vi "generator.vi"() -> ()   [LabVIEW 2009]
uses:
  <vilib>/measure/madcrms.llb/Basic Averaged DC-RMS for N Chan.vi
  <vilib>/measure/matone.llb/Extract Single Tone Information N Chan.vi
  <vilib>/Utility/file.llb/Write To Spreadsheet File (DBL).vi
  <vilib>/measure/NI_MAPro.lvlib
  <vilib>/Analysis/NI_AALPro.lvlib
panel:
  out "Fuel GPM":dbl
  in  "Clear Data":bool
  in  "Record Data":bool
  in  "Save Data To CSV?":bool
  in  "CSV Save Path":path
  in  "Append?":bool
  out "Shop Water\nFlow (GPM)":dbl
  out "Jacket \nWater\nFlow\n(GPM)":dbl
  out "Exhaust Temp. (F)":dbl
  out "Shop\nWater\nOut (F)":dbl
  out "Shop\nWater\nIn (F)":dbl
  out "Jacket\nWater\nOut (F)":dbl
  out "Jacket \nWater\nIn (F)":dbl
  out "Oil Temp. (F)":dbl
  out "Fuel (gal.)":dbl(slide) scale=0.0..20.0
  out "Load (kW)":dbl format="%.1f"
  in  "?":bool
  # "CSV Headers:\ntime [s],\nT oil [F],\nT jacket in [F] ,\nT jacket out [F],\nT shop in [F],\nT shop out [F],\nT exhaust [F],\nLoad [kW],\nFuel [gal] ,\nShop Flow [GPM],\nJacket Flow [GPM]"
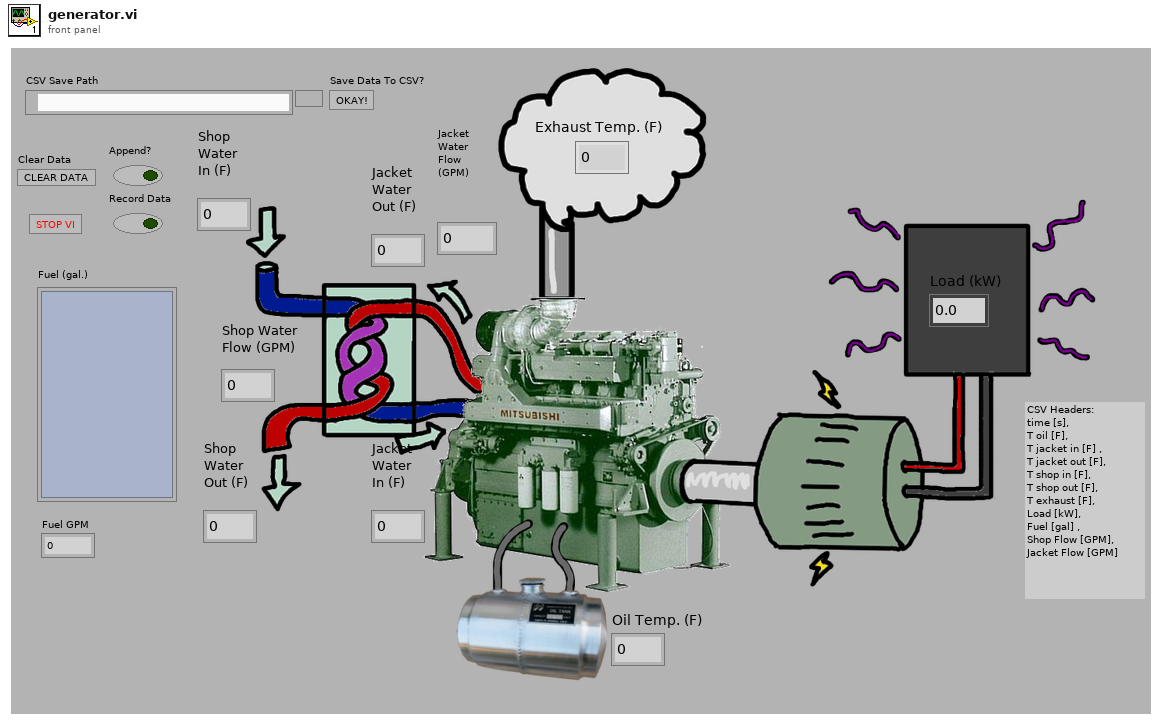
[diagram p1: front panel]
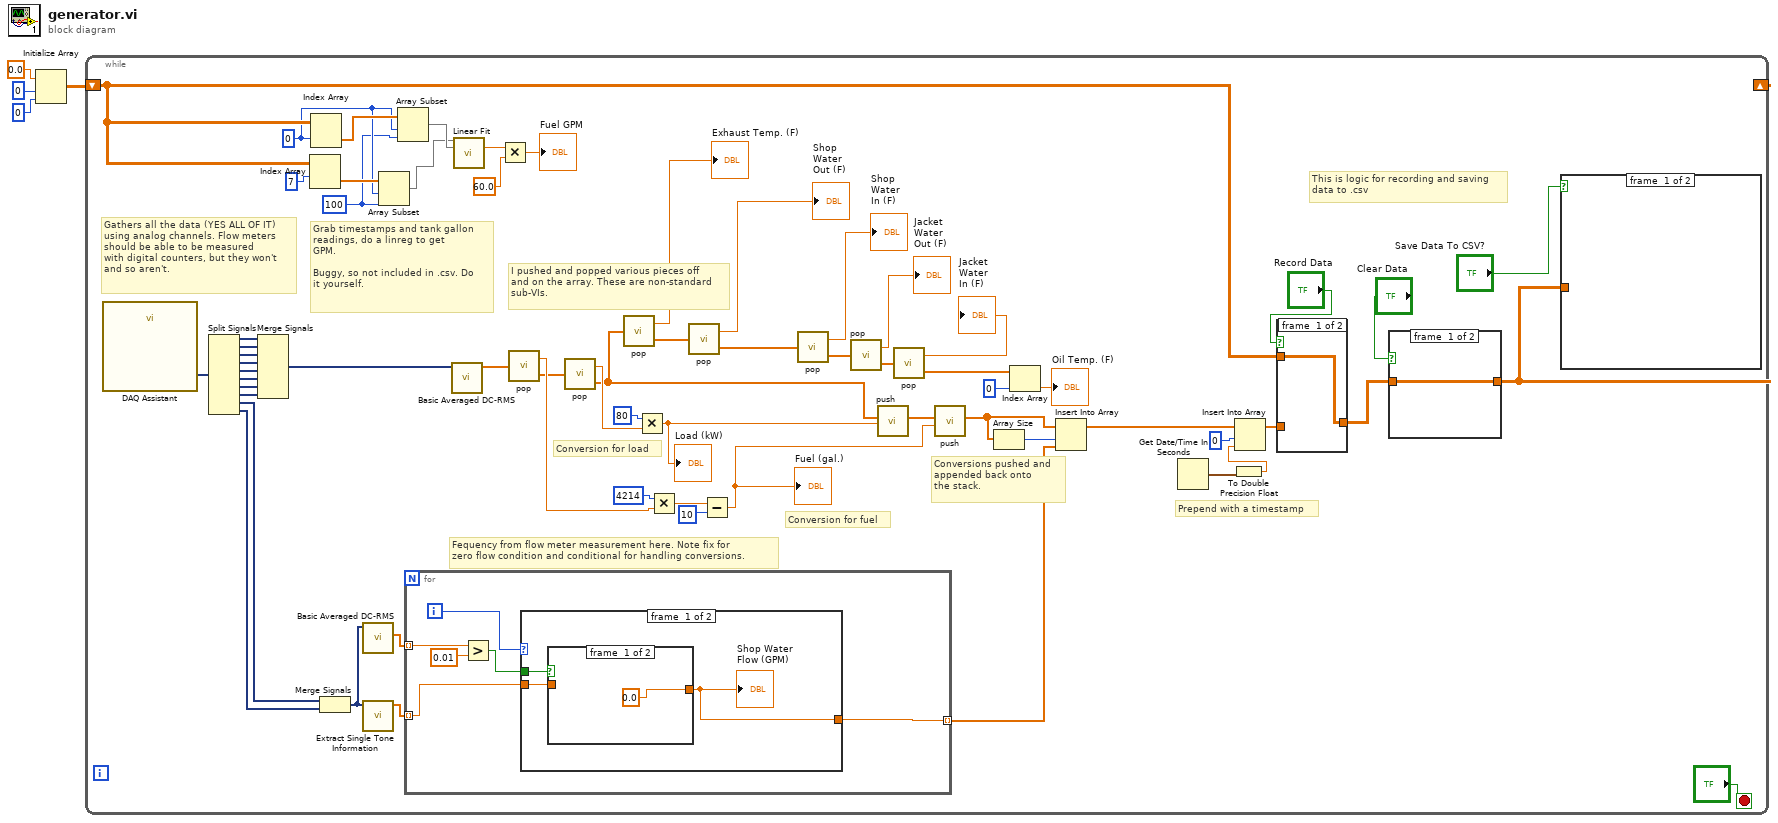
[diagram p0: block diagram]
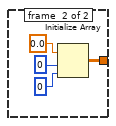
[diagram p2: hidden frame]
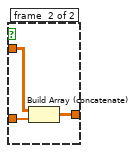
[diagram p3: hidden frame]
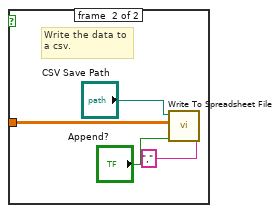
[diagram p4: hidden frame]
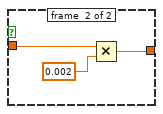
[diagram p5: hidden frame]
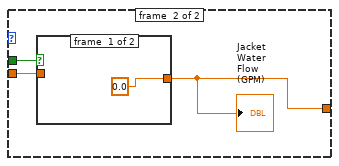
[diagram p6: hidden frame]
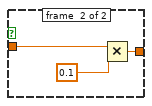
[diagram p7: hidden frame]
diagram:
  n1 = Initialize Array(0.0, 0, 0) -> (w1:dbl[][])
  n2 = while {
    shift-right: [w21] -> _
    shift-left: w1 -> [w16]
    stop <- "?" stop-if-true
    w8 = 100
    w10 = 0
    # "Grab timestamps and tank gallon\nreadings, do a linreg to get\nGPM.\n\nBuggy, so not included in .csv. Do\nit yourself."
    # "This is logic for recording and saving\ndata to .csv"
    # "Conversions pushed and\nappended back onto\nthe stack."
    # "Conversion for fuel"
    # "Conversion for load"
    # "I pushed and popped various pieces off\nand on the array. These are non-standard\nsub-VIs."
    # "Fequency from flow meter measurement here. Note fix for\nzero flow condition and conditional for handling conversions."
    # "Gathers all the data (YES ALL OF IT)\nusing analog channels. Flow meters\nshould be able to be measured\nwith digital counters, but they won't\nand so aren't."
    # "Prepend with a timestamp"
    n3 = call "DAQ Assistant"() -> ("data"=w55:dynamicdata)  [unwired: 17 in, 2 out]
    n4 = Split Signals(w55) -> (w42:dynamicdata, w41:dynamicdata, w40:dynamicdata, w39:dynamicdata, w38:dynamicdata, w37:dynamicdata, w36:dynamicdata, w35:dynamicdata, w34:dynamicdata, w33:dynamicdata)  [unwired: 10 in]
    n5 = Merge Signals(w42, w41, w40, w39, w38, w37, w36, w35) -> (w44:dynamicdata)
    n6 = Index Array(array=w16, index (row)=7) -> (element=w14:dbl[])  [unwired: 1 in]
    n7 = Index Array(array=w16, index (row)=w10) -> (element=w13:dbl[])  [unwired: 1 in]
    n8 = Merge Signals(w34, w33) -> (w43:dynamicdata)
    n9 = call-poly <vilib>:"Basic Averaged DC-RMS.vi"("signals in"=w43) -> ("RMS values"=w45:dbl[])  [unwired: 7 in, 3 out]
    n10 = call-poly <vilib>:"Extract Single Tone Information.vi"("time signals in"=w43) -> ("detected frequencies"=w46:dbl[])  [unwired: 5 in, 5 out]
    n11 = Array Subset(array=w14, index=w10, length=w8) -> (w11:dbl[])
    n12 = Array Subset(array=w13, index=w10, length=w8) -> (w12:dbl[])
    n13 = for {
      tunnel: w46 -> [w82] mode=indexing
      tunnel: w45 -> [w87] mode=indexing
      tunnel: [w84] -> w17 mode=indexing
      i -> [w85]
      n14 = Greater?(x=w87, y=0.01) -> (0:w83:bool)
      n15 = case shown="0, Default" w85 {
        tunnel: [w89 w95] -> w84
        tunnel: w83 -> [w90 w97]
        tunnel: w82 -> [w88 w96]
        frame #0 {
          n16 = case shown="False" w90 {
            tunnel: [0.0 w93] -> w89
            tunnel: w88 -> [_ w92]
            frame #0 {
            }
            frame #1 {
              n17 = Multiply(x=w92, y=0.002) -> (x*y=w93:dbl)
            }
          }
          "Shop Water\nFlow (GPM)" <- w89
        }
        frame #1 {
          n18 = case shown="False" w97 {
            tunnel: [0.0 w100] -> w95
            tunnel: w96 -> [_ w99]
            frame #0 {
            }
            frame #1 {
              n19 = Multiply(x=w99, y=0.1) -> (x*y=w100:dbl)
            }
          }
          "Jacket \nWater\nFlow\n(GPM)" <- w95
        }
      }
    }
    n20 = call-poly <vilib>:"Basic Averaged DC-RMS.vi"("signals in"=w44) -> ("DC values"=w52:dbl[])  [unwired: 7 in, 3 out]
    n21 = call <vilib>:"Linear Fit.vi"("Y"=w11, "X"=w12) -> ("slope"=w6:dbl)  [unwired: 9 in, 4 out]
    n22 = Multiply(x=w6, y=60.0) -> (x*y=→"Fuel GPM":dbl)
    n23 = call "pop.vi"("Before"=w52) -> ("Popped"=w53:dbl, "After"=w51:dbl[])  [unwired: 4 in]
    n24 = call "pop.vi"("Before"=w51) -> ("Popped"=w54:dbl, "After"=w26:dbl[])  [unwired: 4 in]
    n25 = call "pop.vi"("Before"=w26) -> ("Popped"=→"Exhaust Temp. (F)":dbl, "After"=w66:dbl[])  [unwired: 4 in]
    n26 = Multiply(x=80, y=w54) -> (x*y=w25:dbl)
    "Load (kW)" <- w25
    n27 = Multiply(x=4214, y=w53) -> (x*y=w50:dbl)
    n28 = call "pop.vi"("Before"=w66) -> ("Popped"=→"Shop\nWater\nOut (F)":dbl, "After"=w64:dbl[])  [unwired: 4 in]
    n29 = Subtract(x=w50, y=10) -> (x-y=w23:dbl)
    "Fuel (gal.)" <- w23
    n30 = call "pop.vi"("Before"=w64) -> ("Popped"=→"Shop\nWater\nIn (F)":dbl, "After"=w62:dbl[])  [unwired: 4 in]
    n31 = call "pop.vi"("Before"=w62) -> ("Popped"=→"Jacket\nWater\nOut (F)":dbl, "After"=w60:dbl[])  [unwired: 4 in]
    n32 = call "push.vi"("Push"=w25, "Before"=w26) -> ("After"=w24:dbl[])  [unwired: 9 in]
    n33 = call "pop.vi"("Before"=w60) -> ("Popped"=→"Jacket \nWater\nIn (F)":dbl, "After"=w58:dbl[])  [unwired: 4 in]
    n34 = call "push.vi"("Push"=w23, "Before"=w24) -> ("After"=w19:dbl[])  [unwired: 9 in]
    n35 = Array Size(array=w19) -> (size(s)=w18:i32)
    n36 = Index Array(array=w58, index=0) -> (element=→"Oil Temp. (F)":dbl)
    n37 = Insert Into Array(array=w19, index=w18, new element=w17) -> (w5:dbl[])
    n38 = Get Date/Time In Seconds() -> (seconds since 1Jan1904=w28:timestamp)
    n39 = To Double Precision Float(number=w28) -> (double precision float=w27:dbl)
    n40 = Insert Into Array(array=w5, index=0, new element=w27) -> (w22:dbl[])
    n41 = case shown="True" "Record Data" {
      tunnel: w22 -> [_ w77]
      tunnel: w16 -> [w74 w76]
      tunnel: [w74 w75] -> w29
      frame #0 {
      }
      frame #1 {
        n42 = Build Array (concatenate)(w76, w77) -> (w75:dbl[][])
      }
    }
    n43 = case shown="True" "Clear Data" {
      tunnel: w29 -> [w69 _]
      tunnel: [w69 w70] -> w21
      frame #0 {
      }
      frame #1 {
        n44 = Initialize Array(0.0, 0, 0) -> (w70:dbl[][])
      }
    }
    n45 = case shown="True" "Save Data To CSV?" {
      tunnel: w21 -> [_ w79]
      frame #0 {
      }
      frame #1 {
        # "Write the data to\na csv."
        n46 = call-poly <vilib>:"Write To Spreadsheet File.vi"("delimiter (\\t)"=",", "append to file? (new file:F)"="Append?", "2D data"=w79, "file path (dialog if empty)"="CSV Save Path") -> ()  [unwired: 4 in, 1 out]
      }
    }
  }
